vi "Read Ini.vi"(8 "error in (no error)":errorcluster, 10 "key":string="key", 11 "section":string="Section") -> (0 "error out":errorcluster, 3 "value":string)   [LabVIEW 2020]
uses:
  <vilib>/Utility/config.llb/Read Key (String).vi
  <vilib>/Utility/config.llb/NI_LVConfig.lvlib
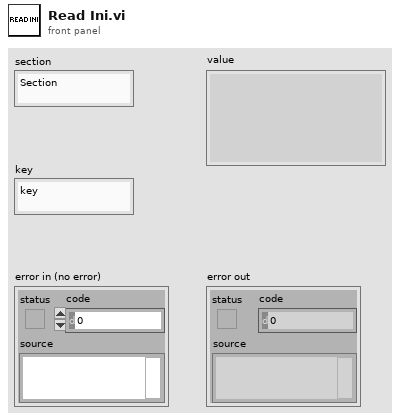
[diagram p1: front panel]
types:
  T1 = typedef "NI_LVConfig.lvlib/Config Data RefNum.ctl" = refnum<k1>
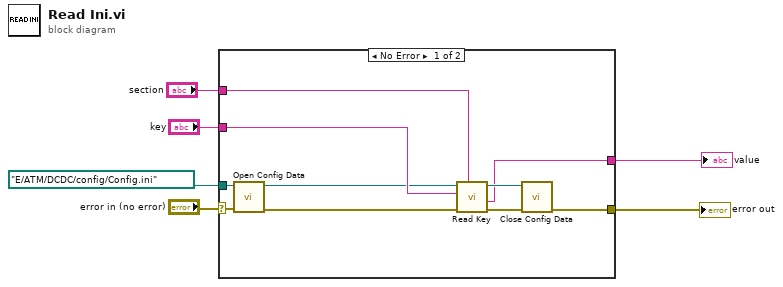
[diagram p0: block diagram]
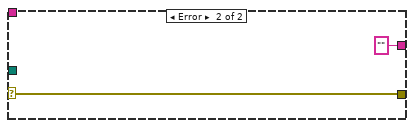
[diagram p2: hidden frame]
diagram:
  n1 = case shown="No Error" "error in (no error)" {
    selector: "error in (no error)" -> [w11 w18]
    tunnel: "key" -> [w16 _]
    tunnel: "section" -> [w13 _]
    tunnel: path "E:/ATM/DCDC/config/Config.ini" ("appended path") -> [w12 _]
    tunnel: [w8 w18] -> w3
    tunnel: [w7 "" ("value")] -> w2
    frame No Error {
      n2 = call <vilib>:"Open Config Data.vi"("error in (no error)"=w11, "configuration file path"=w12) -> ("error out"=w15:errorcluster, "refnum"=w14:T1)  [unwired: 7 in, 1 out]
      n3 = call-poly <vilib>:"Read Key.vi"("section"=w13, "error in (no error)"=w15, "key"=w16, "refnum"=w14) -> ("error out"=w10:errorcluster, "value"=w7:string, "refnum out"=w9:T1)  [unwired: 4 in, 1 out]
      n4 = call <vilib>:"Close Config Data.vi"("error in (no error)"=w10, "refnum"=w9) -> ("error out"=w8:errorcluster)  [unwired: 8 in, 1 out]
    }
    frame Error {
    }
  }
  "error out" <- w3
  "value" <- w2
